vi "drawString.vi"(0 "reference":refnum<class "Graphics.lvclass">, 1 "text":string, 2 "textPos":T4 {"y" format="%.2f"; "x" format="%.2f"}, 3 "fontType":T3, 4 "font":T2, 5 "error in (no error)":errorcluster, 7 "alignment(left, top)":T1) -> (14 "reference out":refnum<class "Graphics.lvclass">, 19 "error out":errorcluster)   [LabVIEW 2014, in "Graphics.lvclass"]
doc: "Draw a string"
uses:
  <resource>/Framework/Providers/Open_GDS/UML/Graphics_class/Graphics.lvclass
  <resource>/Framework/Providers/Open_GDS/UML/General/Point/Point Point2D.ctl
  <resource>/Framework/Providers/Open_GDS/UML/Graphics_class/LvFontType.ctl
  <resource>/Framework/Providers/Open_GDS/UML/Graphics_class/FontType.ctl
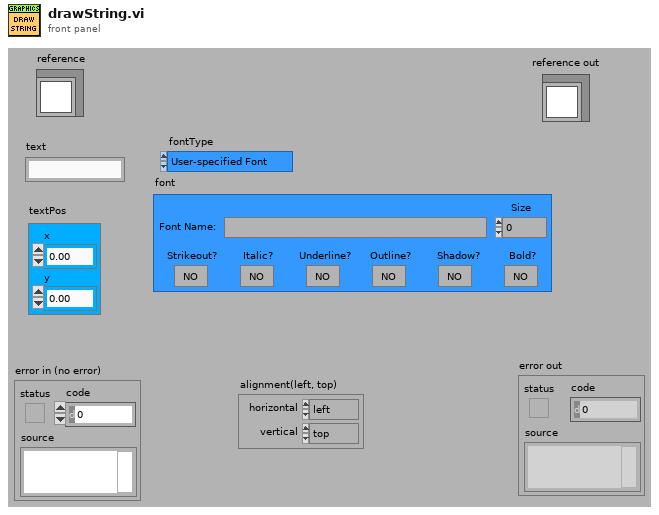
[diagram p1: front panel]
types:
  T1 = cluster{"horizontal":enum16{"left", "center", "right"}, "vertical":enum16{"top", "center", "bottom"}}
  T2 = typedef "Graphics.lvclass/FontType.ctl" = cluster{"Font Name:":string, "Size":i16, "Strikeout?":bool, "Italic?":bool, "Underline?":bool, "Outline?":bool, "Shadow?":bool, "Bold?":bool}
  T3 = typedef "Graphics.lvclass/LvFontType.ctl" = enum16{"User-specified Font", "Application Font", "System Font", "Dialog Font"}
  T4 = typedef "Point Point2D.ctl" = cluster{"x":dbl, "y":dbl}
  T5 = typedef "Graphics.lvclass/ObjectAttributes.ctl" = cluster{"drawColor":u32, "backgroundColor":u32, "font":T2, "fontType":T3, "picture":picture, "stroke":T6, "scaleX":dbl, "scaleY":dbl, "screenRef":refnum<vi>, "offsetX":dbl, "offsetY":dbl}
  T6 = typedef "Graphics.lvclass/StrokeType.ctl" = enum16{"USE_DEFAULT", "SOLID", "DOTTED"}
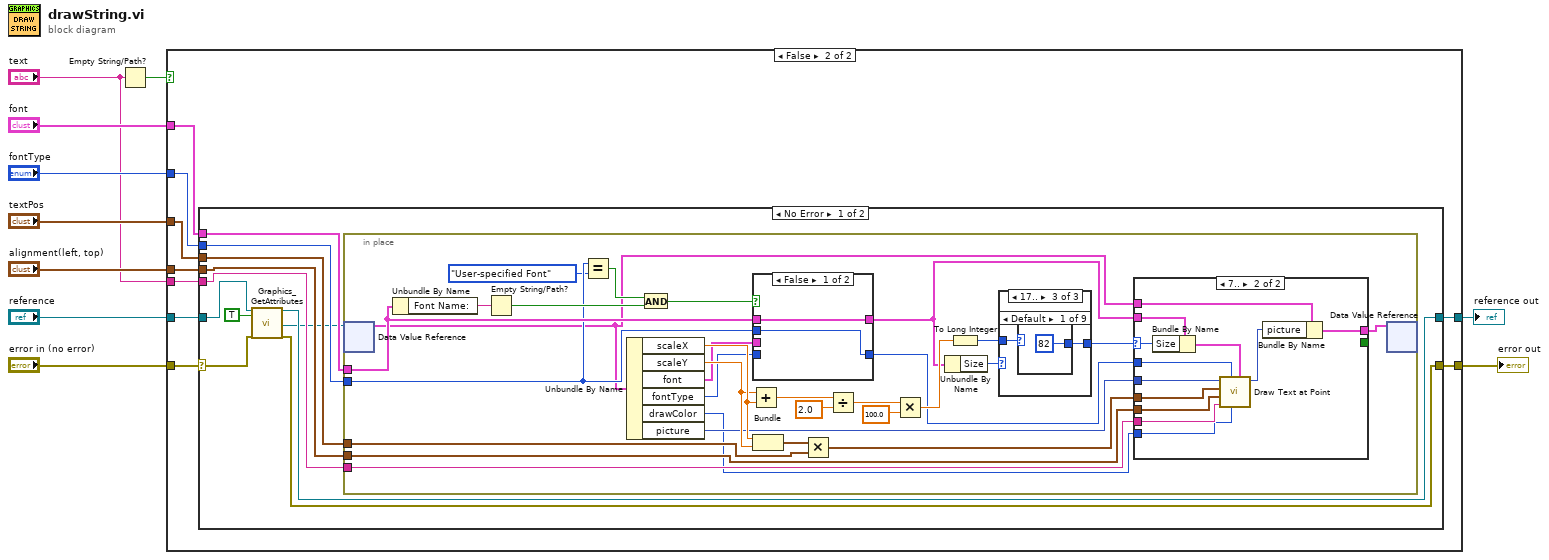
[diagram p0: block diagram]
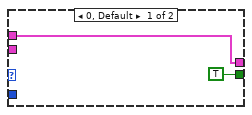
[diagram p3: hidden frame]
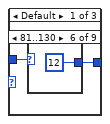
[diagram p4: hidden frame]
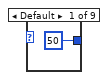
[diagram p5: hidden frame]
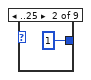
[diagram p6: hidden frame]
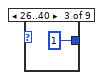
[diagram p7: hidden frame]
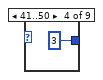
[diagram p8: hidden frame]
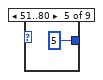
[diagram p9: hidden frame]
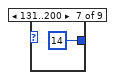
[diagram p10: hidden frame]
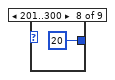
[diagram p11: hidden frame]
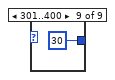
[diagram p12: hidden frame]
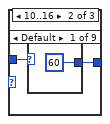
[diagram p13: hidden frame]
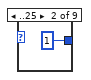
[diagram p14: hidden frame]
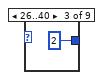
[diagram p15: hidden frame]
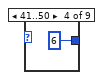
[diagram p16: hidden frame]
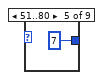
[diagram p17: hidden frame]
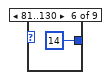
[diagram p18: hidden frame]
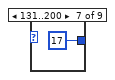
[diagram p19: hidden frame]
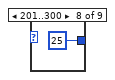
[diagram p20: hidden frame]
diagram:
  n1 = Empty String/Path?(string/path="text") -> (empty?=w1:bool)
  n2 = case shown="False" w1 {
    tunnel: "error in (no error)" -> [w11 w21]
    tunnel: "reference" -> [w12 w20]
    tunnel: [w11 w19] -> w8
    tunnel: [w12 w18] -> w7
    tunnel: "textPos" -> [_ w17]
    tunnel: "fontType" -> [_ w16]
    tunnel: "font" -> [_ w15]
    tunnel: "alignment(left, top)" -> [_ w14]
    tunnel: "text" -> [_ w13]
    frame True {
    }
    frame False {
      n3 = case shown="No Error" w21 {
        selector: w21 -> [w32 w114]
        tunnel: w20 -> [w31 w115]
        tunnel: [w23 w114] -> w19
        tunnel: [w30 w115] -> w18
        tunnel: w13 -> [w25 _]
        tunnel: w17 -> [w27 _]
        tunnel: w16 -> [w28 _]
        tunnel: w15 -> [w29 _]
        tunnel: w14 -> [w24 _]
        frame No Error {
          n4 = call <resource>:"Graphics_GetAttributes.vi"("reference in"=w31, "OnlyGetDvrReference(False)"=TRUE, "error in (no error)"=w32) -> ("reference out"=w30:refnum<class "Graphics.lvclass">, "DataRef"=w22:refnum<data-value>, "error out"=w23:errorcluster)  [unwired: 13 in, 1 out]
          n5 = in-place {
            in-place-border: w29 -> [w59]
            in-place-border: w28 -> [w58]
            in-place-border: w27 -> [w55]
            in-place-border: w25 -> [w45]
            in-place-border: w24 -> [w42]
            n6 = in-place-dvr #1(w22) -> (w34:T5)  [unwired: 1 out]
            n7 = Unbundle By Name(w59) -> ("Font Name:"=w62:string)
            n8 = Empty String/Path?(string/path=w62) -> (empty?=w60:bool)
            n9 = Equal?(x=w58, y=LvFontType."User-specified Font" ("fontType")) -> (x = y?=w61:bool)
            n10 = Unbundle By Name(w34) -> ("scaleX"=w40:dbl, "scaleY"=w39:dbl, "font"=w38:T2, "fontType"=w37:T3, "drawColor"=w35:u32, "picture"=w36:picture)
            n11 = And(x=w61, y=w60) -> (x .and. y?=w57:bool)
            n12 = Add(x=w39, y=w40) -> (x+y=w54:dbl)
            n13 = case shown="False" w57 {
              tunnel: w38 -> [_ w112]
              tunnel: w37 -> [_ w113]
              tunnel: [w110 w113] -> w44
              tunnel: [w111 w112] -> w43
              tunnel: w59 -> [w111 _]
              tunnel: w58 -> [w110 _]
              frame False {
              }
              frame True {
              }
            }
            n14 = Bundle("scaleX"=w40, "scaleY"=w39) -> (w56:cluster{"scaleX":dbl, "scaleY":dbl})  [unwired: 1 out]
            n15 = Multiply(x=w56, y=w55) -> (x*y=w41:T4)
            n16 = Divide(x=w54, y=2.0) -> (x/y=w51:dbl)
            n17 = Multiply(x=w51, y=100.0) -> (x*y=w49:dbl)
            n18 = Unbundle By Name(w43) -> ("Size"=w52:i16)
            n19 = To Long Integer(number=w49) -> (32bit integer=w48:i32)
            n20 = case shown="17.." w52 {
              tunnel: [w78 w89 w99] -> w46
              tunnel: w48 -> [w77 w88 w100]
              frame Default {
                n21 = case shown="81..130" w77 {
                  tunnel: [i16 50 ("Size 9") i16 1 ("Size") i16 1 ("Size 2") i16 3 ("Size 3") i16 5 ("Size 4") i16 12 ("Size 5") i16 14 ("Size 6") i16 20 ("Size 7") i16 30 ("Size 8")] -> w78
                  frame Default {
                  }
                  frame ..25 {
                  }
                  frame 26..40 {
                  }
                  frame 41..50 {
                  }
                  frame 51..80 {
                  }
                  frame 81..130 {
                  }
                  frame 131..200 {
                  }
                  frame 201..300 {
                  }
                  frame 301..400 {
                  }
                }
              }
              frame 10..16 {
                n22 = case shown="Default" w88 {
                  tunnel: [i16 60 ("Size 9") i16 1 ("Size") i16 2 ("Size 2") i16 6 ("Size 3") i16 7 ("Size 4") i16 14 ("Size 5") i16 17 ("Size 6") i16 25 ("Size 7") i16 40 ("Size 8")] -> w89
                  frame Default {
                  }
                  frame ..25 {
                  }
                  frame 26..40 {
                  }
                  frame 41..50 {
                  }
                  frame 51..80 {
                  }
                  frame 81..130 {
                  }
                  frame 131..200 {
                  }
                  frame 201..300 {
                  }
                  frame 301..400 {
                  }
                }
              }
              frame 17.. {
                n23 = case shown="Default" w100 {
                  tunnel: [i16 82 ("Size") i16 2 ("Size") i16 5 ("Size") i16 7 ("Size") i16 12 ("Size") i16 18 ("Size") i16 26 ("Size") i16 36 ("Size") i16 55 ("Size")] -> w99
                  frame Default {
                  }
                  frame ..25 {
                  }
                  frame 26..40 {
                  }
                  frame 41..50 {
                  }
                  frame 51..80 {
                  }
                  frame 81..130 {
                  }
                  frame 131..200 {
                  }
                  frame 201..300 {
                  }
                  frame 301..400 {
                  }
                }
              }
            }
            n24 = case shown="7.." w46 {
              selector: w46 -> [_ w65]
              tunnel: w34 -> [w64 w76]
              tunnel: [w64 w75] -> w33
              tunnel: w36 -> [_ w74]
              tunnel: w45 -> [_ w72]
              tunnel: w35 -> [_ w71]
              tunnel: w44 -> [_ w70]
              tunnel: w43 -> [_ w69]
              tunnel: w42 -> [_ w67]
              tunnel: w41 -> [_ w66]
              tunnel: [TRUE _] -> _
              frame 0, Default {
              }
              frame 7.. {
                n25 = Bundle By Name(cluster=w69, "Size"=w65) -> (w68:T2)
                n26 = call <vilib>:"Draw Text at Point.vi"("[user-specified font]"=w68, "text color(black)"=w71, "desired font(Application)"=w70, "text"=w72, "alignment(left, top)"=w67, "origin"=w66, "picture"=w74) -> ("new picture"=w73:picture)  [unwired: 2 in, 2 out]
                n27 = Bundle By Name(cluster=w76, "picture"=w73) -> (w75:T5)
              }
            }
            n28 = in-place-dvr #1(w33) -> ()  [unwired: 2 out]
          }
        }
        frame Error {
        }
      }
    }
  }
  "reference out" <- w7
  "error out" <- w8
